vi "EventDetectionMode vol no 6230 DO.vi"(8 "error in (no error)":errorcluster, 11 "SetupInfo_IN":T1={"ConfigParameters_Analog"={"JAI camera fps"=240.0, "Bi-Lateral Galvo xy scan range (V)"=0.7, "Bi-Lateral Galvo xy scan frequency (Hz)"=500, "AOM Blind percent (%)"=0.1, "AOM start blind percent (%) "=70.0, "ROI threshold"=1.0, "AO Sampling rate"=1000000.0}, "ConfigParameters_Digital"={"Steps per volume"=25.0, "Time per volume (s)"=0.4, "OG start layer"=15.0, "Objective Lin Rising Vel (micron/ms）"=1.0, "Image depth (micron)"=200.0, "OG latency (s)"=10.0, "OG repitation"=3.0, "OG end layer"=17.0, "Shock1 duration (s)"=0.001, "Shock2 duration (s)"=0.001, "Shock3 duration (s)"=0.01, "Shock4 duration (s)"=0.01, "Shock5 duration (s)"=0.1, "Shock duration_New"=[]}, "ConfigParameters_Other1"={"Frontal Galvo xy scan range (V)"=0.14, "Frontal Galvo xy scan frequency (Hz)"=500, "PFI 0 digital clock frequency"=500000.0, "Window size for layer index"=0.5, "sCMOS fps"=95.0}, "ConfigParameters_Others2"={"#Trials baseline"=6, "#Trials test"=6, "Time before acq. (s)"=360.0, "Time before test (s)"=600.0, "#Blocks acquisition"=5, "Inter-trial interval baseline (s)"=60.0, "#Trials per acquition block"=6, "Inter-block interval acquisition (s)"=360.0, "Inter-trial interval acquisition (s)"=20.0, "Flash latency (s)"=10.0, "Flash duration (s)"=3.2, "Response duration (s)"=10.0, "MaxTimeEventDetection (s)"=6, "StimType"=enum."Flash", "#MaxEvents"=6}, "ProcessParametersOut"={"stand Z vol Acquisition time (s)"=0.2631578947368421, "stand Z vol Backward time (s)"=0.13684210526315793, "Objective scan volt"=5.0, "Bi-lateral Galvo Z scan volt"=0.1800000180000018, "Frontal Galvo Z scan volt"=0.14940000509752818, "Objective step length (micron)"=8.0, "OG Z volet Linear Dec time (s)"=0.024, "OG Z vol Stim. steps time (s)"=0.031578947368421054, "OG Z vol Linear Acc time (s)"=0.112, "#Vol. of flash"=8, "#Vol. of shock"=1, "#Vol. bef flash"=25, "#Vol. aft flash"=17, "OG Z vol Linear Dec time (s)"=0.112, "OG Z vol time (s)"=0.39073684210526316, "Stack duration"=[0.001, 0.001, 0.01, 0.01, 0.1], "AOM stand. value size"=400000, "Plane indexing length"=0, "#Vol. blank"=0, "#Vol. blank before acq"=1000000, "#Vol. blank before test"=263158, " #Inter-block interval acquisition (Ed-St Vol)"=1000000}, "WaveformParameters"={"stand Z vol Acquisition samp info"={"Fs"=1000000.0, "#s"=263158.0}, "stand Z vol Backward samp info"={"Fs"=1000000.0, "#s"=136842.0}, "OG Z vol Linear Acc samp info"={"Fs"=1000000.0, "#s"=112000.0}, "OG Z vol Stim. steps samp info"={"Fs"=1000000.0, "#s"=31579.0}, "OG Z volet Linear Dec samp info"={"Fs"=1000000.0, "#s"=24000.0}, "OG Z vol Linear Dec samp info"={"Fs"=1000000.0, "#s"=112000.0}, "OG Z vol samp info"={"Fs"=1000000.0, "#s"=390737.0}, "stand Z vol backforth samp info"={"Fs"=1000000.0, "#s"=400000.0}}, "AnalogWaveform"={"Bi-lateral Galvo Z stand waveform"={"t0"=timestamp(0 s since 1904-01-01), "dt"=1.0, "Y"=[]}, "Frontal Galvo Z stand waveform"={"t0"=timestamp(0 s since 1904-01-01), "dt"=1.0, "Y"=[]}, "Bi-lateral Galvo XY stand waveform"={"t0"=timestamp(0 s since 1904-01-01), "dt"=1.0, "Y"=[]}, "Frontal Galvo XY stand waveform"={"t0"=timestamp(0 s since 1904-01-01), "dt"=1.0, "Y"=[]}, "sCMOS stand waveform"={"t0"=timestamp(0 s since 1904-01-01), "dt"=1.0, "Y"=[]}, "Detection objective stand waveform"={"t0"=timestamp(0 s since 1904-01-01), "dt"=1.0, "Y"=[]}, "AOM stand waveform"={"t0"=timestamp(0 s since 1904-01-01), "dt"=1.0, "Y"=[]}, "PFI 0 clock stand waveform"={"t0"=timestamp(0 s since 1904-01-01), "dt"=1.0, "Y"=[]}, "Bi-lateral Galvo Z OG waveform"={"t0"=timestamp(0 s since 1904-01-01), "dt"=1.0, "Y"=[]}, "Bi-lateral Galvo XY OG waveform"={"t0"=timestamp(0 s since 1904-01-01), "dt"=1.0, "Y"=[]}, "Frontal Galvo Z OG waveform"={"t0"=timestamp(0 s since 1904-01-01), "dt"=1.0, "Y"=[]}, "Frontal Galvo XY OG waveform"={"t0"=timestamp(0 s since 1904-01-01), "dt"=1.0, "Y"=[]}, "sCMOS OG waveform"={"t0"=timestamp(0 s since 1904-01-01), "dt"=1.0, "Y"=[]}, "Detection objective OG waveform"={"t0"=timestamp(0 s since 1904-01-01), "dt"=1.0, "Y"=[]}, "AOM OG waveform"={"t0"=timestamp(0 s since 1904-01-01), "dt"=1.0, "Y"=[]}, "PFI 0 clock OG wavee"={"t0"=timestamp(0 s since 1904-01-01), "dt"=1.0, "Y"=[]}, "sCMOS blank waveform"={"t0"=timestamp(0 s since 1904-01-01), "dt"=1.0, "Y"=[]}, "All analog OG wave"=[], "All analog stand wave"=[], "All analog blank wave"=[], "BufferWaveform_Analog"=[], "Bi-lateral Galvo Z XY"={"t0"=timestamp(0 s since 1904-01-01), "dt"=1.0, "Y"=[]}, "Frontal Galvo Z XY"={"t0"=timestamp(0 s since 1904-01-01), "dt"=1.0, "Y"=[]}, "sCMOS Trigger XY"={"t0"=timestamp(0 s since 1904-01-01), "dt"=1.0, "Y"=[]}, "Detection objective XY"={"t0"=timestamp(0 s since 1904-01-01), "dt"=1.0, "Y"=[]}, "AOM XY"={"t0"=timestamp(0 s since 1904-01-01), "dt"=1.0, "Y"=[]}, "Analog_XY"=[]}, "DigitalWaveform"={"AllDigitalStandWave"=[], "AllDigialEvokedWave"=[], "AllDigialOGWave"=[], "AllDigitalPairWave_1"=[], "AllDigitalPairWave_2"=[], "AllDigitalPairWave_3"=[], "AllDigitalPairWave_4"=[], "AllDigitalPairWave_5"=[], "Plane Indexing"={"t0"=timestamp(0 s since 1904-01-01), "dt"=0.0, "Y"={"transitions"=[], "data"=[]}, "error"={"status"=FALSE, "code"=37421928, "source"=""}}, "Plane indexing P0.5 OG"={"t0"=timestamp(0 s since 1904-01-01), "dt"=0.0, "Y"={"transitions"=[], "data"=[]}, "error"={"status"=FALSE, "code"=37421928, "source"=""}}, "AllDigitalPairWaves"=[], "BufferWaveform_Digital"=[], "AllDigitalBlankWave"=[], "Digial_XY"=[], "Digital_XY_flash"=[], "Digial_XY DMD"=[]}, "PhysicalResource"={"PhysicalChannels_AI"="", "PhysicalChannels_AO"="", "PhysicalChannels_DO"="", "Task_AnalogOutput"="", "Task_DigitalOutput"="", "Task_AnalogInput"=""}, "ControlsRef"={"Mode_1"=refnum, "EventDetectionMode"=refnum, "Mode_2A"=refnum, "StimulationMode"=refnum, "Mode_2B"=refnum, "ErrorMeg"=refnum}, "test"=""} {"ConfigParameters_Other1"."Frontal Galvo xy scan frequency (Hz)" min=500 max=500; "ConfigParameters_Other1"."Frontal Galvo xy scan range (V)" min=0.0 max=1.5; "ConfigParameters_Analog"."AOM start blind percent (%)" min=10.0 max=90.0; "ConfigParameters_Analog"."AOM Blind percent (%)" min=0.1 max=100.0; "ConfigParameters_Analog"."Bi-Lateral Galvo xy scan frequency (Hz)" min=500 max=500; "ConfigParameters_Analog"."Bi-Lateral Galvo xy scan range (V)" min=0.0 max=1.5}) -> (0 "error out":errorcluster, 3 "SetupInfo_OUT":T1={"ConfigParameters_Analog"={"JAI camera fps"=240.0, "Bi-Lateral Galvo xy scan range (V)"=0.7, "Bi-Lateral Galvo xy scan frequency (Hz)"=500, "AOM Blind percent (%)"=0.1, "AOM start blind percent (%) "=70.0, "ROI threshold"=1.0, "AO Sampling rate"=1000000.0}, "ConfigParameters_Digital"={"Steps per volume"=25.0, "Time per volume (s)"=0.4, "OG start layer"=15.0, "Objective Lin Rising Vel (micron/ms）"=1.0, "Image depth (micron)"=200.0, "OG latency (s)"=10.0, "OG repitation"=3.0, "OG end layer"=17.0, "Shock1 duration (s)"=0.001, "Shock2 duration (s)"=0.001, "Shock3 duration (s)"=0.01, "Shock4 duration (s)"=0.01, "Shock5 duration (s)"=0.1, "Shock duration_New"=[]}, "ConfigParameters_Other1"={"Frontal Galvo xy scan range (V)"=0.14, "Frontal Galvo xy scan frequency (Hz)"=500, "PFI 0 digital clock frequency"=500000.0, "Window size for layer index"=0.5, "sCMOS fps"=95.0}, "ConfigParameters_Others2"={"#Trials baseline"=6, "#Trials test"=6, "Time before acq. (s)"=360.0, "Time before test (s)"=600.0, "#Blocks acquisition"=5, "Inter-trial interval baseline (s)"=60.0, "#Trials per acquition block"=6, "Inter-block interval acquisition (s)"=360.0, "Inter-trial interval acquisition (s)"=20.0, "Flash latency (s)"=10.0, "Flash duration (s)"=3.2, "Response duration (s)"=10.0, "MaxTimeEventDetection (s)"=6, "StimType"=enum."Flash", "#MaxEvents"=6}, "ProcessParametersOut"={"stand Z vol Acquisition time (s)"=0.2631578947368421, "stand Z vol Backward time (s)"=0.13684210526315793, "Objective scan volt"=5.0, "Bi-lateral Galvo Z scan volt"=0.1800000180000018, "Frontal Galvo Z scan volt"=0.14940000509752818, "Objective step length (micron)"=8.0, "OG Z volet Linear Dec time (s)"=0.024, "OG Z vol Stim. steps time (s)"=0.031578947368421054, "OG Z vol Linear Acc time (s)"=0.112, "#Vol. of flash"=8, "#Vol. of shock"=1, "#Vol. bef flash"=25, "#Vol. aft flash"=17, "OG Z vol Linear Dec time (s)"=0.112, "OG Z vol time (s)"=0.39073684210526316, "Stack duration"=[0.001, 0.001, 0.01, 0.01, 0.1], "AOM stand. value size"=400000, "Plane indexing length"=0, "#Vol. blank"=0, "#Vol. blank before acq"=1000000, "#Vol. blank before test"=263158, " #Inter-block interval acquisition (Ed-St Vol)"=1000000}, "WaveformParameters"={"stand Z vol Acquisition samp info"={"Fs"=1000000.0, "#s"=263158.0}, "stand Z vol Backward samp info"={"Fs"=1000000.0, "#s"=136842.0}, "OG Z vol Linear Acc samp info"={"Fs"=1000000.0, "#s"=112000.0}, "OG Z vol Stim. steps samp info"={"Fs"=1000000.0, "#s"=31579.0}, "OG Z volet Linear Dec samp info"={"Fs"=1000000.0, "#s"=24000.0}, "OG Z vol Linear Dec samp info"={"Fs"=1000000.0, "#s"=112000.0}, "OG Z vol samp info"={"Fs"=1000000.0, "#s"=390737.0}, "stand Z vol backforth samp info"={"Fs"=1000000.0, "#s"=400000.0}}, "AnalogWaveform"={"Bi-lateral Galvo Z stand waveform"={"t0"=timestamp(0 s since 1904-01-01), "dt"=1.0, "Y"=[]}, "Frontal Galvo Z stand waveform"={"t0"=timestamp(0 s since 1904-01-01), "dt"=1.0, "Y"=[]}, "Bi-lateral Galvo XY stand waveform"={"t0"=timestamp(0 s since 1904-01-01), "dt"=1.0, "Y"=[]}, "Frontal Galvo XY stand waveform"={"t0"=timestamp(0 s since 1904-01-01), "dt"=1.0, "Y"=[]}, "sCMOS stand waveform"={"t0"=timestamp(0 s since 1904-01-01), "dt"=1.0, "Y"=[]}, "Detection objective stand waveform"={"t0"=timestamp(0 s since 1904-01-01), "dt"=1.0, "Y"=[]}, "AOM stand waveform"={"t0"=timestamp(0 s since 1904-01-01), "dt"=1.0, "Y"=[]}, "PFI 0 clock stand waveform"={"t0"=timestamp(0 s since 1904-01-01), "dt"=1.0, "Y"=[]}, "Bi-lateral Galvo Z OG waveform"={"t0"=timestamp(0 s since 1904-01-01), "dt"=1.0, "Y"=[]}, "Bi-lateral Galvo XY OG waveform"={"t0"=timestamp(0 s since 1904-01-01), "dt"=1.0, "Y"=[]}, "Frontal Galvo Z OG waveform"={"t0"=timestamp(0 s since 1904-01-01), "dt"=1.0, "Y"=[]}, "Frontal Galvo XY OG waveform"={"t0"=timestamp(0 s since 1904-01-01), "dt"=1.0, "Y"=[]}, "sCMOS OG waveform"={"t0"=timestamp(0 s since 1904-01-01), "dt"=1.0, "Y"=[]}, "Detection objective OG waveform"={"t0"=timestamp(0 s since 1904-01-01), "dt"=1.0, "Y"=[]}, "AOM OG waveform"={"t0"=timestamp(0 s since 1904-01-01), "dt"=1.0, "Y"=[]}, "PFI 0 clock OG wavee"={"t0"=timestamp(0 s since 1904-01-01), "dt"=1.0, "Y"=[]}, "sCMOS blank waveform"={"t0"=timestamp(0 s since 1904-01-01), "dt"=1.0, "Y"=[]}, "All analog OG wave"=[], "All analog stand wave"=[], "All analog blank wave"=[], "BufferWaveform_Analog"=[], "Bi-lateral Galvo Z XY"={"t0"=timestamp(0 s since 1904-01-01), "dt"=1.0, "Y"=[]}, "Frontal Galvo Z XY"={"t0"=timestamp(0 s since 1904-01-01), "dt"=1.0, "Y"=[]}, "sCMOS Trigger XY"={"t0"=timestamp(0 s since 1904-01-01), "dt"=1.0, "Y"=[]}, "Detection objective XY"={"t0"=timestamp(0 s since 1904-01-01), "dt"=1.0, "Y"=[]}, "AOM XY"={"t0"=timestamp(0 s since 1904-01-01), "dt"=1.0, "Y"=[]}, "Analog_XY"=[]}, "DigitalWaveform"={"AllDigitalStandWave"=[], "AllDigialEvokedWave"=[], "AllDigialOGWave"=[], "AllDigitalPairWave_1"=[], "AllDigitalPairWave_2"=[], "AllDigitalPairWave_3"=[], "AllDigitalPairWave_4"=[], "AllDigitalPairWave_5"=[], "Plane Indexing"={"t0"=timestamp(0 s since 1904-01-01), "dt"=0.0, "Y"={"transitions"=[], "data"=[]}, "error"={"status"=FALSE, "code"=37421928, "source"=""}}, "Plane indexing P0.5 OG"={"t0"=timestamp(0 s since 1904-01-01), "dt"=0.0, "Y"={"transitions"=[], "data"=[]}, "error"={"status"=FALSE, "code"=37421928, "source"=""}}, "AllDigitalPairWaves"=[], "BufferWaveform_Digital"=[], "AllDigitalBlankWave"=[], "Digial_XY"=[], "Digital_XY_flash"=[], "Digial_XY DMD"=[]}, "PhysicalResource"={"PhysicalChannels_AI"="", "PhysicalChannels_AO"="", "PhysicalChannels_DO"="", "Task_AnalogOutput"="", "Task_DigitalOutput"="", "Task_AnalogInput"=""}, "ControlsRef"={"Mode_1"=refnum, "EventDetectionMode"=refnum, "Mode_2A"=refnum, "StimulationMode"=refnum, "Mode_2B"=refnum, "ErrorMeg"=refnum}, "test"=""} {"ConfigParameters_Other1"."Frontal Galvo xy scan frequency (Hz)" min=500 max=500; "ConfigParameters_Other1"."Frontal Galvo xy scan range (V)" min=0.0 max=1.5; "ConfigParameters_Analog"."AOM start blind percent (%)" min=10.0 max=90.0; "ConfigParameters_Analog"."AOM Blind percent (%)" min=0.1 max=100.0; "ConfigParameters_Analog"."Bi-Lateral Galvo xy scan frequency (Hz)" min=500 max=500; "ConfigParameters_Analog"."Bi-Lateral Galvo xy scan range (V)" min=0.0 max=1.5})   [LabVIEW 2018]
uses:
  SetupInfo.ctl
  ConfigParameters_Analog.ctl
  ConfigParameters_Digital.ctl
  ConfigParameters_Others1.ctl
  ConfigParameters_Others2.ctl
  ProcessParametersOut.ctl
  WaveformParameters.ctl
  AnalogWaveform.ctl
  DigitalWaveform.ctl
  PhysicalResource.ctl
  ControlsRef.ctl
  <vilib>/Analysis/baseanly.llb/Mean (DBL).vi
  Trigger_Global.vi
  <vilib>/Analysis/NI_AALBase.lvlib
panel:
  out "OG?":bool
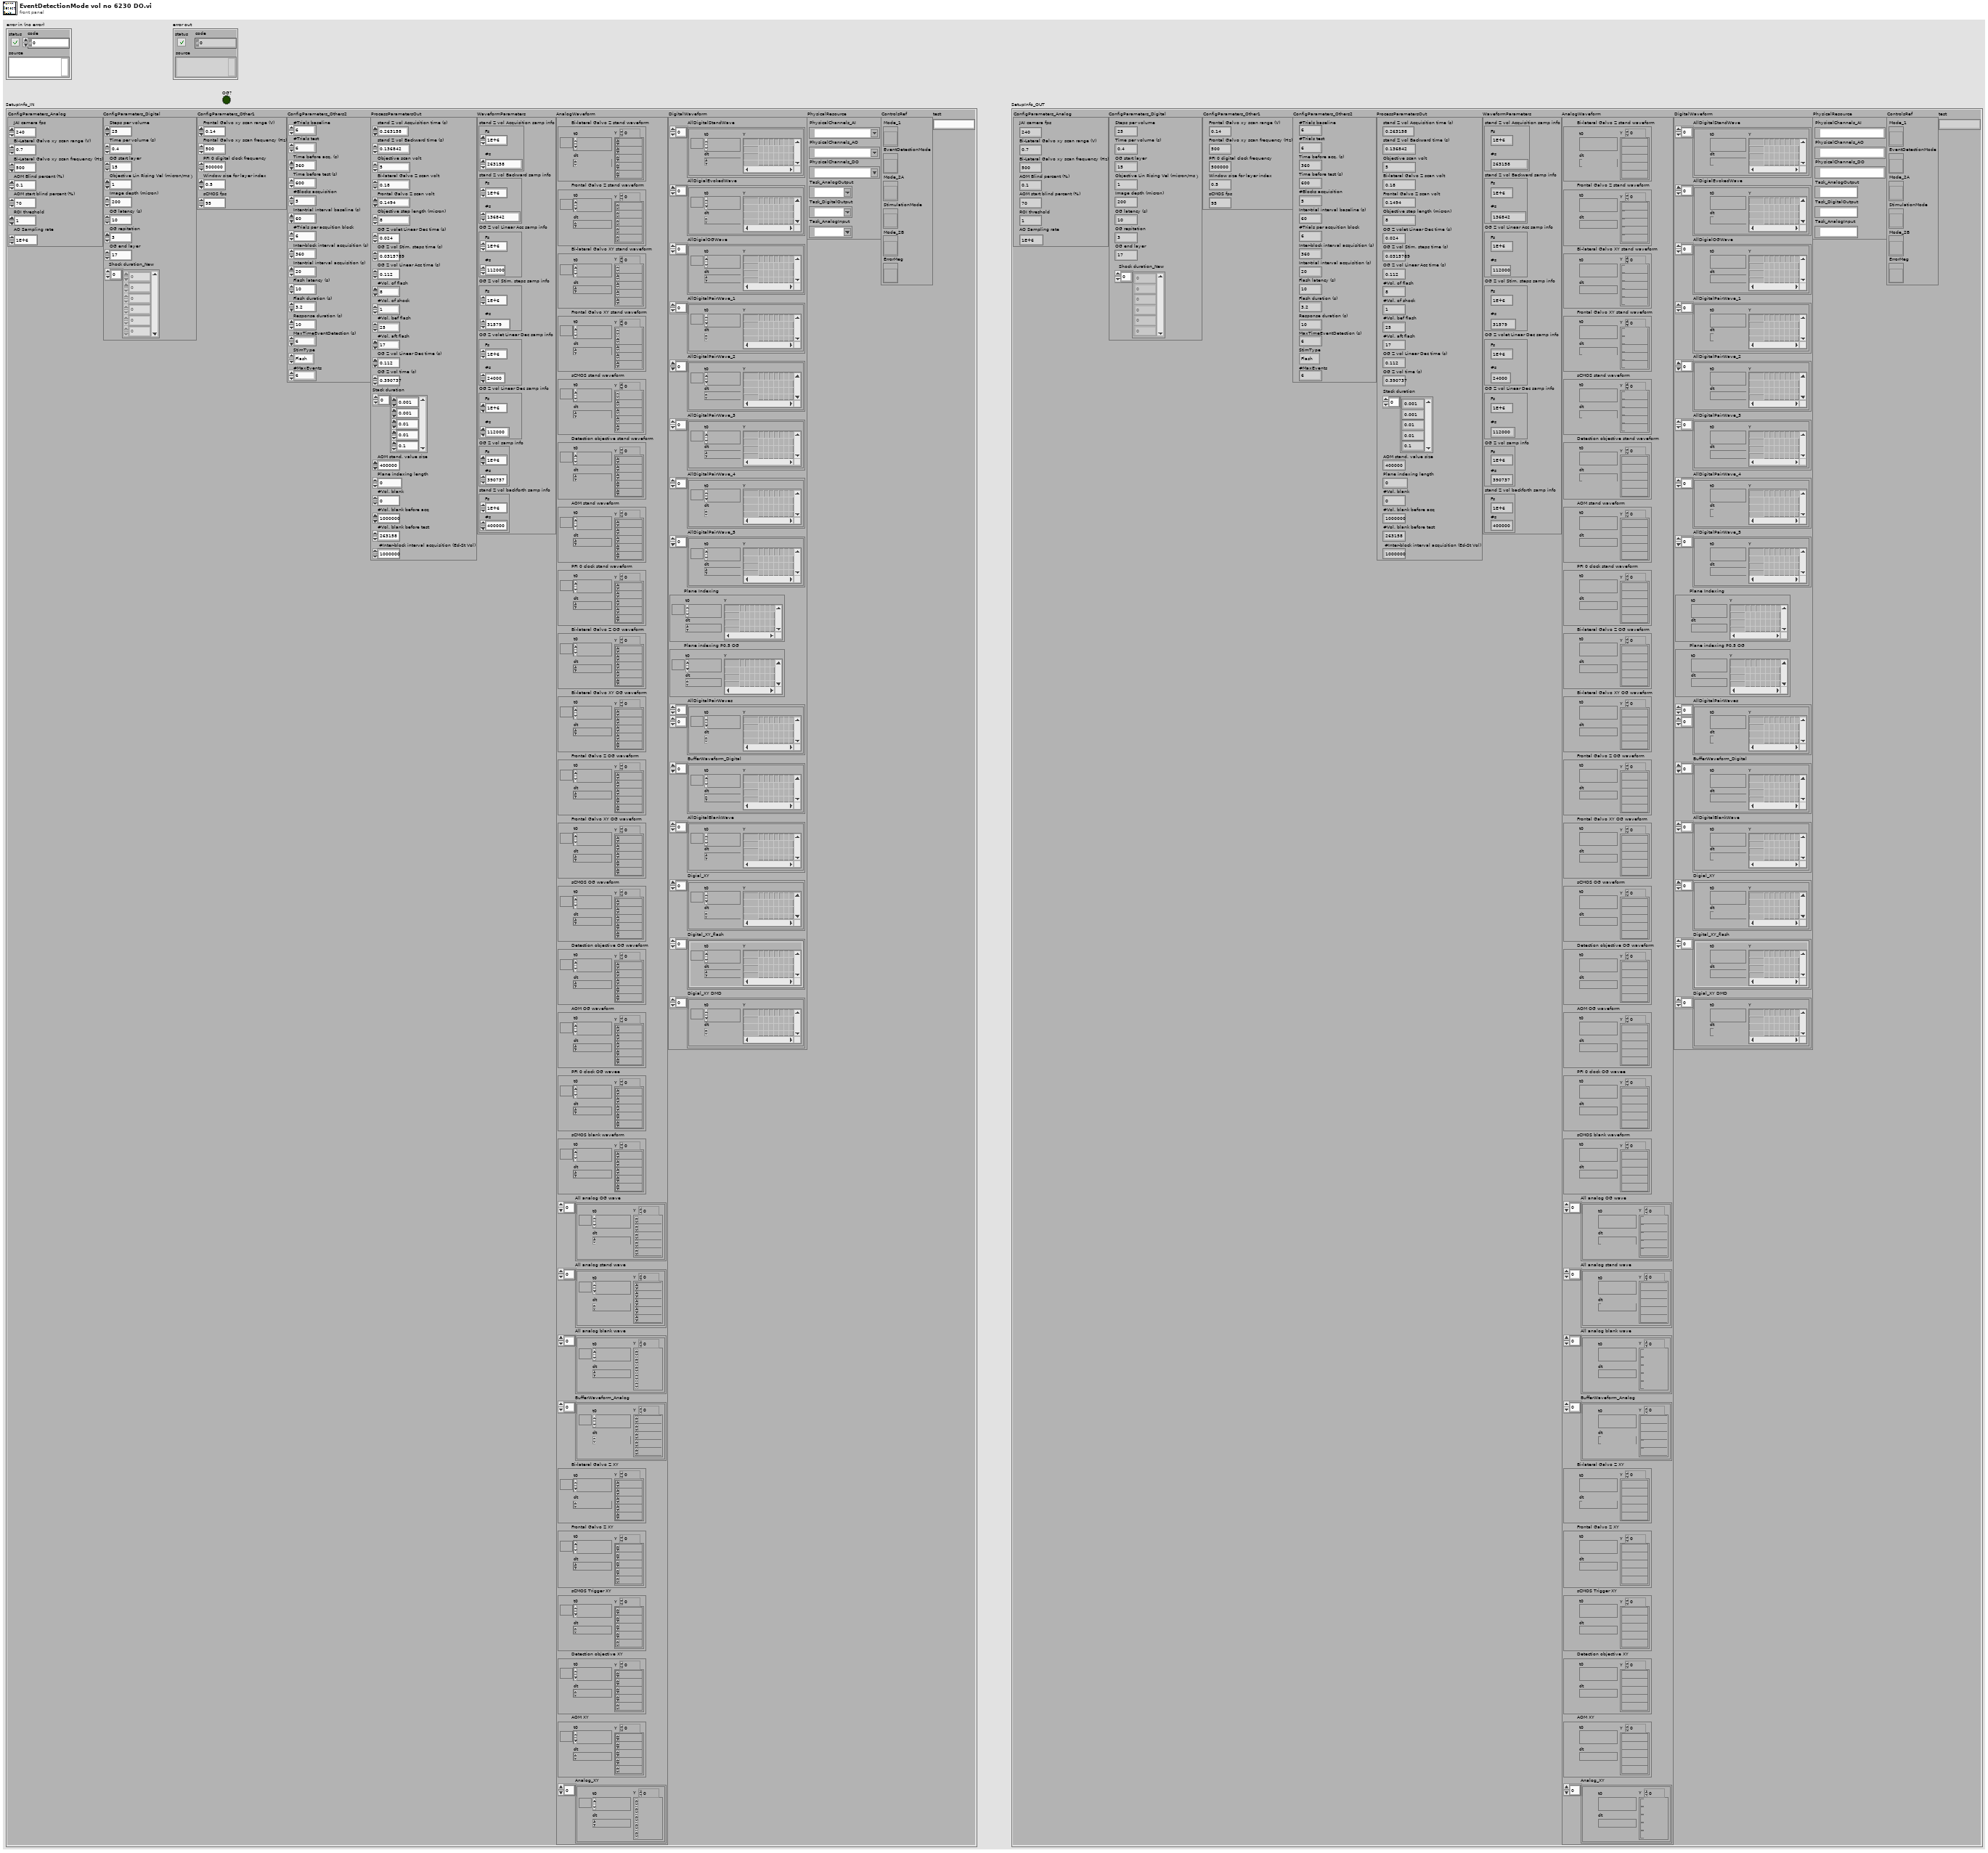
[diagram p1: front panel]
types:
  T1 = typedef "SetupInfo.ctl" = cluster{"ConfigParameters_Analog":T2, "ConfigParameters_Digital":T3, "ConfigParameters_Other1":T4, "ConfigParameters_Others2":T5, "ProcessParametersOut":T6, "WaveformParameters":T7, "AnalogWaveform":T8, "DigitalWaveform":T9, "PhysicalResource":T10, "ControlsRef":T11, "test":string}
  T2 = typedef "ConfigParameters_Analog.ctl" = cluster{"JAI camera fps":dbl, "Bi-Lateral Galvo xy scan range (V)":dbl, "Bi-Lateral Galvo xy scan frequency (Hz)":i16, "AOM Blind percent (%)":dbl, "AOM start blind percent (%) ":dbl, "ROI threshold":dbl, "AO Sampling rate":dbl}
  T3 = typedef "ConfigParameters_Digital.ctl" = cluster{"Steps per volume":dbl, "Time per volume (s)":dbl, "OG start layer":dbl, "Objective Lin Rising Vel (micron/ms）":dbl, "Image depth (micron)":dbl, "OG latency (s)":dbl, "OG repitation":dbl, "OG end layer":dbl, "Shock1 duration (s)":dbl, "Shock2 duration (s)":dbl, "Shock3 duration (s)":dbl, "Shock4 duration (s)":dbl, "Shock5 duration (s)":dbl, "Shock duration_New":dbl[]}
  T4 = typedef "ConfigParameters_Others1.ctl" = cluster{"Frontal Galvo xy scan range (V)":dbl, "Frontal Galvo xy scan frequency (Hz)":i16, "PFI 0 digital clock frequency":dbl, "Window size for layer index":dbl, "sCMOS fps":dbl}
  T5 = typedef "ConfigParameters_Others2.ctl" = cluster{"#Trials baseline":i32, "#Trials test":i32, "Time before acq. (s)":dbl, "Time before test (s)":dbl, "#Blocks acquisition":i32, "Inter-trial interval baseline (s)":dbl, "#Trials per acquition block":i32, "Inter-block interval acquisition (s)":dbl, "Inter-trial interval acquisition (s)":dbl, "Flash latency (s)":dbl, "Flash duration (s)":dbl, "Response duration (s)":dbl, "MaxTimeEventDetection (s)":i32, "StimType":enum16{"Flash", "OG"}, "#MaxEvents":i32}
  T6 = typedef "ProcessParametersOut.ctl" = cluster{"stand Z vol Acquisition time (s)":dbl, "stand Z vol Backward time (s)":dbl, "Objective scan volt":dbl, "Bi-lateral Galvo Z scan volt":dbl, "Frontal Galvo Z scan volt":dbl, "Objective step length (micron)":dbl, "OG Z volet Linear Dec time (s)":dbl, "OG Z vol Stim. steps time (s)":dbl, "OG Z vol Linear Acc time (s)":dbl, "#Vol. of flash":i32, "#Vol. of shock":i32, "#Vol. bef flash":i32, "#Vol. aft flash":i32, "OG Z vol Linear Dec time (s)":dbl, "OG Z vol time (s)":dbl, "Stack duration":dbl[], "AOM stand. value size":i32, "Plane indexing length":i32, "#Vol. blank":i32, "#Vol. blank before acq":i32, "#Vol. blank before test":i32, " #Inter-block interval acquisition (Ed-St Vol)":i32}
  T7 = typedef "WaveformParameters.ctl" = cluster{"stand Z vol Acquisition samp info":cluster{"Fs":dbl, "#s":dbl}, "stand Z vol Backward samp info":cluster{"Fs":dbl, "#s":dbl}, "OG Z vol Linear Acc samp info":cluster{"Fs":dbl, "#s":dbl}, "OG Z vol Stim. steps samp info":cluster{"Fs":dbl, "#s":dbl}, "OG Z volet Linear Dec samp info":cluster{"Fs":dbl, "#s":dbl}, "OG Z vol Linear Dec samp info":cluster{"Fs":dbl, "#s":dbl}, "OG Z vol samp info":cluster{"Fs":dbl, "#s":dbl}, "stand Z vol backforth samp info":cluster{"Fs":dbl, "#s":dbl}}
  T8 = typedef "AnalogWaveform.ctl" = cluster{"Bi-lateral Galvo Z stand waveform":waveform(dbl), "Frontal Galvo Z stand waveform":waveform(dbl), "Bi-lateral Galvo XY stand waveform":waveform(dbl), "Frontal Galvo XY stand waveform":waveform(dbl), "sCMOS stand waveform":waveform(dbl), "Detection objective stand waveform":waveform(dbl), "AOM stand waveform":waveform(dbl), "PFI 0 clock stand waveform":waveform(dbl), "Bi-lateral Galvo Z OG waveform":waveform(dbl), "Bi-lateral Galvo XY OG waveform":waveform(dbl), "Frontal Galvo Z OG waveform":waveform(dbl), "Frontal Galvo XY OG waveform":waveform(dbl), "sCMOS OG waveform":waveform(dbl), "Detection objective OG waveform":waveform(dbl), "AOM OG waveform":waveform(dbl), "PFI 0 clock OG wavee":waveform(dbl), "sCMOS blank waveform":waveform(dbl), "All analog OG wave":waveform(dbl)[], "All analog stand wave":waveform(dbl)[], "All analog blank wave":waveform(dbl)[], "BufferWaveform_Analog":waveform(dbl)[], "Bi-lateral Galvo Z XY":waveform(dbl), "Frontal Galvo Z XY":waveform(dbl), "sCMOS Trigger XY":waveform(dbl), "Detection objective XY":waveform(dbl), "AOM XY":waveform(dbl), "Analog_XY":waveform(dbl)[]}
  T9 = typedef "DigitalWaveform.ctl" = cluster{"AllDigitalStandWave":digitalwaveform[], "AllDigialEvokedWave":digitalwaveform[], "AllDigialOGWave":digitalwaveform[], "AllDigitalPairWave_1":digitalwaveform[], "AllDigitalPairWave_2":digitalwaveform[], "AllDigitalPairWave_3":digitalwaveform[], "AllDigitalPairWave_4":digitalwaveform[], "AllDigitalPairWave_5":digitalwaveform[], "Plane Indexing":digitalwaveform, "Plane indexing P0.5 OG":digitalwaveform, "AllDigitalPairWaves":digitalwaveform[][], "BufferWaveform_Digital":digitalwaveform[], "AllDigitalBlankWave":digitalwaveform[], "Digial_XY":digitalwaveform[], "Digital_XY_flash":digitalwaveform[], "Digial_XY DMD":digitalwaveform[]}
  T10 = typedef "PhysicalResource.ctl" = cluster{"PhysicalChannels_AI":tag, "PhysicalChannels_AO":tag, "PhysicalChannels_DO":tag, "Task_AnalogOutput":refnum<k21>, "Task_DigitalOutput":refnum<k21>, "Task_AnalogInput":refnum<k21>}
  T11 = typedef "ControlsRef.ctl" = cluster{"Mode_1":refnum<vi>, "EventDetectionMode":refnum<vi>, "Mode_2A":refnum<vi>, "StimulationMode":refnum<vi>, "Mode_2B":refnum<vi>, "ErrorMeg":refnum<vi>}
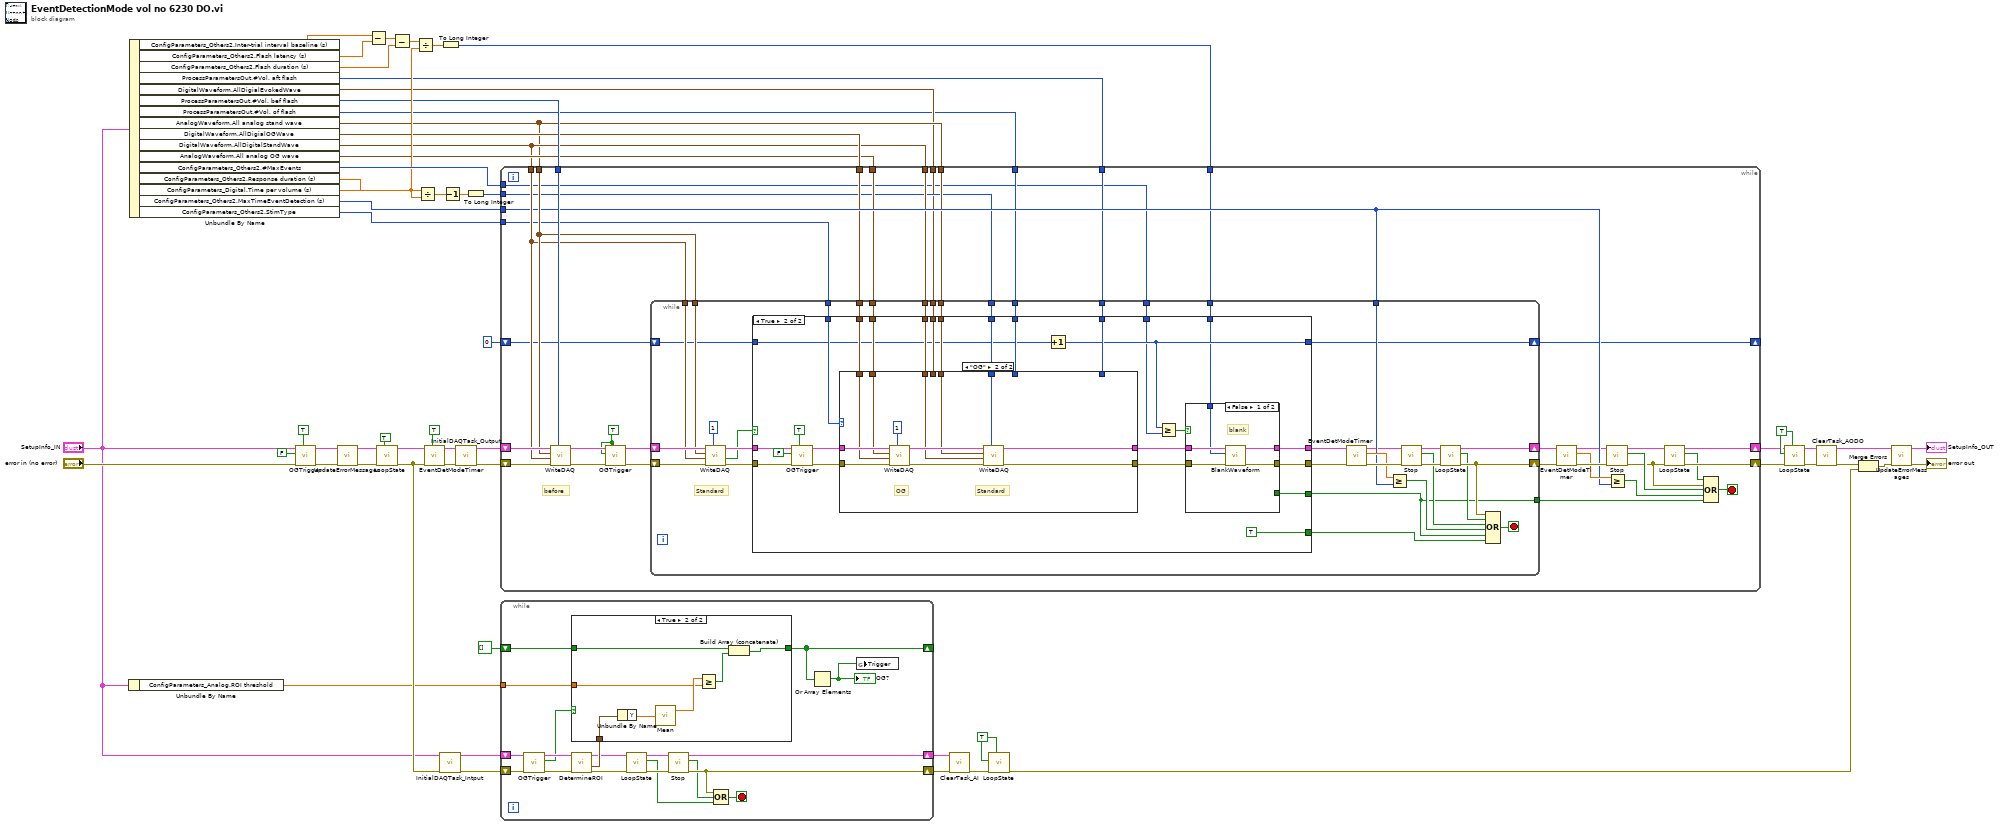
[diagram p0: block diagram]
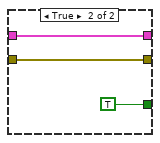
[diagram p3: hidden frame]
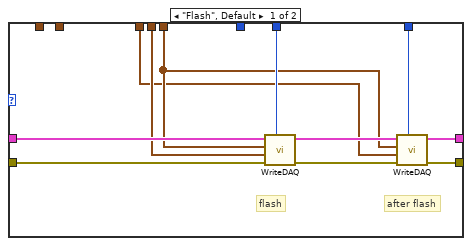
[diagram p4: hidden frame]
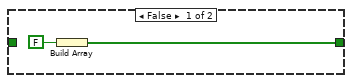
[diagram p5: hidden frame]
diagram:
  w41 = TRUE ("Write?")
  w49 = TRUE ("Write?")
  n1 = Unbundle By Name("SetupInfo_IN") -> ("ConfigParameters_Analog.ROI threshold"=w11:dbl)
  n2 = Unbundle By Name("SetupInfo_IN") -> ("ConfigParameters_Others2.Inter-trial interval baseline (s)"=w28:dbl, "ConfigParameters_Others2.Flash latency (s)"=w27:dbl, "ConfigParameters_Others2.Flash duration (s)"=w25:dbl, "ProcessParametersOut.#Vol. aft flash"=w3:i32, "DigitalWaveform.AllDigialEvokedWave"=w5:digitalwaveform[], "ProcessParametersOut.#Vol. bef flash"=w21:i32, "ProcessParametersOut.#Vol. of flash"=w4:i32, "AnalogWaveform.All analog stand wave"=w6:waveform(dbl)[], "DigitalWaveform.AllDigialOGWave"=w9:digitalwaveform[], "DigitalWaveform.AllDigitalStandWave"=w7:digitalwaveform[], "AnalogWaveform.All analog OG wave"=w8:waveform(dbl)[], "ConfigParameters_Others2.#MaxEvents"=w48:i32, "ConfigParameters_Others2.Response duration (s)"=w47:dbl, "ConfigParameters_Digital.Time per volume (s)"=w23:dbl, "ConfigParameters_Others2.MaxTimeEventDetection (s)"=w43:i32, "ConfigParameters_Others2.StimType"=w32:enum16{"Flash", "OG"})
  n3 = call "OGTrigger.vi"("Write?"=TRUE, "error in (no error)"="error in (no error)", "StateIn"=FALSE) -> ("error out"=w15:errorcluster)  [unwired: 7 in, 1 out]
  n4 = call "UpdateErrorMessages.vi"("error in (no error)"=w15, "SetupInfo_IN"="SetupInfo_IN") -> ("error out"=w33:errorcluster, "SetupInfo_OUT"=w34:T1)  [unwired: 8 in]
  n5 = Subtract(x=w28, y=w27) -> (x-y=w26:dbl)
  n6 = call "LoopState.vi"("Write?"=TRUE, "error in (no error)"=w33) -> ("error out"=w18:errorcluster)  [unwired: 8 in, 1 out]
  n7 = Subtract(x=w26, y=w25) -> (x-y=w24:dbl)
  n8 = Divide(x=w24, y=w23) -> (x/y=w22:dbl)
  n9 = Divide(x=w47, y=w23) -> (x/y=w46:dbl)
  n10 = call "EventDetModeTimer.vi"("Initial"=TRUE, "error in (no error)"=w18) -> ("error out"=w19:errorcluster)  [unwired: 8 in, 1 out]
  n11 = call "InitialDAQTask_Intput.vi"("error in (no error)"=w18, "SetupInfo_IN"="SetupInfo_IN") -> ("error out"=w55:errorcluster, "SetupInfo_OUT"=w42:T1)  [unwired: 8 in]
  n12 = To Long Integer(number=w22) -> (32bit integer=w2:i32)
  n13 = Decrement(x=w46) -> (x-1=w45:dbl)
  n14 = call "InitialDAQTask_Output.vi"("error in (no error)"=w19, "SetupInfo_IN"=w34) -> ("error out"=w17:errorcluster, "SetupInfo_OUT"=w20:T1)  [unwired: 8 in]
  n15 = To Long Integer(number=w45) -> (32bit integer=w31:i32)
  n16 = while {
    shift-right: [w83] -> w29
    shift-left: w17 -> [w80]
    shift-right: [w58] -> w30
    shift-left: w20 -> [w81]
    tunnel: w48 -> [w62]
    tunnel: w31 -> [w66]
    tunnel: w43 -> [w75]
    tunnel: w32 -> [w67]
    tunnel: w21 -> [w79]
    tunnel: w6 -> [w77]
    tunnel: w7 -> [w76]
    tunnel: w9 -> [w71]
    tunnel: w8 -> [w70]
    tunnel: w7 -> [w69]
    tunnel: w6 -> [w68]
    tunnel: w5 -> [w65]
    tunnel: w4 -> [w64]
    tunnel: w3 -> [w63]
    tunnel: w2 -> [w61]
    shift-right: [w60] -> _
    shift-left: 0 -> [w59]
    stop <- w87 stop-if-true
    w74 = TRUE ("Write?")
    # "before"
    n17 = call "WriteDAQ.vi"("Cycle"=w79, "error in (no error)"=w80, "DigitalWaveform_In"=w76, "AnalogWaveform_In"=w77, "SetupInfo_IN"=w81) -> ("error out"=w72:errorcluster, "SetupInfo_OUT"=w78:T1)  [unwired: 4 in, 1 out]
    n18 = call "OGTrigger.vi"("Write?"=w74, "error in (no error)"=w72, "StateIn"=w74) -> ("error out"=w73:errorcluster)  [unwired: 7 in, 1 out]
    n19 = while {
      shift-right: [w97] -> w58
      shift-left: w78 -> [w123]
      shift-right: [w115] -> w56
      shift-left: w73 -> [w111]
      tunnel: w77 -> [w122]
      tunnel: w76 -> [w121]
      tunnel: w75 -> [w116]
      tunnel: w71 -> [w109]
      tunnel: w70 -> [w108]
      tunnel: w69 -> [w106]
      tunnel: w68 -> [w105]
      tunnel: w67 -> [w104]
      tunnel: w66 -> [w103]
      tunnel: w65 -> [w102]
      tunnel: w64 -> [w101]
      tunnel: w63 -> [w100]
      shift-right: [w94] -> w60
      shift-left: w59 -> [w95]
      tunnel: w62 -> [w93]
      tunnel: w61 -> [w92]
      tunnel: [w91] -> w57
      stop <- w120 stop-if-true
      # "Standard"
      n20 = call "WriteDAQ.vi"("Cycle"=1, "error in (no error)"=w111, "DigitalWaveform_In"=w121, "AnalogWaveform_In"=w122, "SetupInfo_IN"=w123) -> ("error out"=w98:errorcluster, "Trigger"=w96:bool, "SetupInfo_OUT"=w107:T1)  [unwired: 4 in]
      n21 = case shown="True" w96 {
        tunnel: w109 -> [_ w151]
        tunnel: w108 -> [_ w150]
        tunnel: w107 -> [w125 w149]
        tunnel: w106 -> [_ w148]
        tunnel: w105 -> [_ w147]
        tunnel: w104 -> [_ w146]
        tunnel: w103 -> [_ w145]
        tunnel: w102 -> [_ w144]
        tunnel: w101 -> [_ w143]
        tunnel: w100 -> [_ w142]
        tunnel: [w126 w135] -> w99
        tunnel: w98 -> [w126 w129]
        tunnel: [w125 w136] -> w97
        tunnel: w95 -> [w124 w141]
        tunnel: [w124 w140] -> w94
        tunnel: w93 -> [_ w139]
        tunnel: w92 -> [_ w133]
        tunnel: [_ w132] -> w91
        tunnel: [_ TRUE] -> w90
        frame False {
        }
        frame True {
          n22 = call "OGTrigger.vi"("Write?"=TRUE, "error in (no error)"=w129, "StateIn"=FALSE) -> ("error out"=w128:errorcluster)  [unwired: 7 in, 1 out]
          n23 = case shown="\"OG\"" w146 {
            tunnel: w128 -> [w169 w182]
            tunnel: w149 -> [w170 w181]
            tunnel: [w164 w172] -> w138
            tunnel: [w163 w171] -> w137
            tunnel: w150 -> [_ w180]
            tunnel: w151 -> [_ w179]
            tunnel: w147 -> [w161 w175]
            tunnel: w144 -> [w168 _]
            tunnel: w145 -> [_ w173]
            tunnel: w148 -> [w160 w174]
            tunnel: w143 -> [w167 _]
            tunnel: w142 -> [w162 _]
            frame "Flash", Default {
              # "after flash"
              # "flash"
              n24 = call "WriteDAQ.vi"("Cycle"=w167, "error in (no error)"=w169, "DigitalWaveform_In"=w168, "AnalogWaveform_In"=w161, "SetupInfo_IN"=w170) -> ("error out"=w165:errorcluster, "SetupInfo_OUT"=w166:T1)  [unwired: 4 in, 1 out]
              n25 = call "WriteDAQ.vi"("Cycle"=w162, "error in (no error)"=w165, "DigitalWaveform_In"=w160, "AnalogWaveform_In"=w161, "SetupInfo_IN"=w166) -> ("error out"=w163:errorcluster, "SetupInfo_OUT"=w164:T1)  [unwired: 4 in, 1 out]
            }
            frame "OG" {
              # "Standard"
              # "OG"
              n26 = call "WriteDAQ.vi"("Cycle"=1, "error in (no error)"=w182, "DigitalWaveform_In"=w179, "AnalogWaveform_In"=w180, "SetupInfo_IN"=w181) -> ("error out"=w176:errorcluster, "SetupInfo_OUT"=w177:T1)  [unwired: 4 in, 1 out]
              n27 = call "WriteDAQ.vi"("Cycle"=w173, "error in (no error)"=w176, "DigitalWaveform_In"=w174, "AnalogWaveform_In"=w175, "SetupInfo_IN"=w177) -> ("error out"=w171:errorcluster, "SetupInfo_OUT"=w172:T1)  [unwired: 4 in, 1 out]
            }
          }
          n28 = Increment(x=w141) -> (x+1=w140:i32)
          n29 = Greater Or Equal?(x=w140, y=w139) -> (x >= y?=w134:bool)
          n30 = case shown="False" w134 {
            tunnel: w137 -> [w156 w158]
            tunnel: w138 -> [w155 w159]
            tunnel: [w154 w159] -> w136
            tunnel: [w153 w158] -> w135
            tunnel: w133 -> [w152 _]
            tunnel: [_ TRUE] -> w132
            frame False {
              # "blank"
              n31 = call "BlankWaveform.vi"("error in (no error)"=w156, "Cycle"=w152, "SetupInfo_IN"=w155) -> ("error out"=w153:errorcluster, "SetupInfo_OUT"=w154:T1)  [unwired: 7 in]
            }
            frame True {
            }
          }
        }
      }
      n32 = call "EventDetModeTimer.vi"("error in (no error)"=w99) -> ("error out"=w118:errorcluster, "TimerOut(s)"=w117:dbl)  [unwired: 9 in]
      n33 = Greater Or Equal?(x=w117, y=w116) -> (x >= y?=w112:bool)
      n34 = call "Stop.vi"("error in (no error)"=w118) -> ("error out"=w119:errorcluster, "StateOut"=w113:bool)  [unwired: 9 in]
      n35 = call "LoopState.vi"("error in (no error)"=w119) -> ("error out"=w115:errorcluster, "StateOut"=w114:bool)  [unwired: 9 in]
      n36 = Compound Arithmetic op=OR(w115, w114, w113, w112, w91, w90) -> (w120:bool)
    }
    n37 = call "EventDetModeTimer.vi"("error in (no error)"=w56) -> ("error out"=w88:errorcluster, "TimerOut(s)"=w86:dbl)  [unwired: 9 in]
    n38 = call "Stop.vi"("error in (no error)"=w88) -> ("error out"=w84:errorcluster, "StateOut"=w89:bool)  [unwired: 9 in]
    n39 = Greater Or Equal?(x=w86, y=w75) -> (x >= y?=w85:bool)
    n40 = call "LoopState.vi"("error in (no error)"=w84) -> ("error out"=w83:errorcluster, "StateOut"=w82:bool)  [unwired: 9 in]
    n41 = Compound Arithmetic op=OR(w82, w84, w89, w85, w57) -> (w87:bool)
  }
  n42 = while {
    shift-right: [w198] -> w54
    shift-left: w55 -> [w190]
    shift-right: [w192] -> w53
    shift-left: w42 -> [w188]
    shift-right: [w185] -> _
    shift-left: bool[] [] -> [w187]
    tunnel: w11 -> [w186]
    stop <- w196 stop-if-true
    n43 = call "OGTrigger.vi"("error in (no error)"=w190) -> ("error out"=w191:errorcluster, "StateOut"=w184:bool)  [unwired: 9 in]
    n44 = call "DetermineROI.vi"("error in (no error)"=w191, "SetupInfo_IN"=w188) -> ("error out"=w189:errorcluster, "data"=w193:waveform(dbl), "SetupInfo_OUT"=w192:T1)  [unwired: 7 in]
    n45 = case shown="True" w184 {
      tunnel: w193 -> [_ w201]
      tunnel: [w199 w202] -> w185
      tunnel: w187 -> [_ w205]
      tunnel: w186 -> [_ w203]
      frame False {
        n46 = Build Array(FALSE) -> (w199:bool[])
      }
      frame True {
        n47 = Unbundle By Name(w201) -> ("Y"=w206:dbl[])
        n48 = call-poly <vilib>:"Mean.vi"("X"=w206) -> ("mean"=w207:dbl)  [unwired: 1 out]
        n49 = Greater Or Equal?(x=w207, y=w203) -> (x >= y?=w204:bool)
        n50 = Build Array (concatenate)(w205, w204) -> (w202:bool[])
      }
    }
    n51 = call "LoopState.vi"("error in (no error)"=w189) -> ("error out"=w195:errorcluster, "StateOut"=w194:bool)  [unwired: 9 in]
    n52 = call "Stop.vi"("error in (no error)"=w195) -> ("error out"=w198:errorcluster, "StateOut"=w197:bool)  [unwired: 9 in]
    n53 = Compound Arithmetic op=OR(w198, w197, w194) -> (w196:bool)
    n54 = Or Array Elements(Boolean array=w185) -> (logical OR=w183:bool)
    "OG?" <- w183
    n55 = global write "Trigger_Global.vi" "Trigger"(w183) -> ()
  }
  n56 = call "ClearTask_AI.vi"("error in (no error)"=w54, "SetupInfo_IN"=w53) -> ("error out"=w40:errorcluster)  [unwired: 8 in, 1 out]
  n57 = call "LoopState.vi"("Write?"=w41, "error in (no error)"=w40, "StateIn"=w41) -> ("error out"=w39:errorcluster)  [unwired: 7 in, 1 out]
  n58 = call "LoopState.vi"("Write?"=w49, "error in (no error)"=w29, "StateIn"=w49) -> ("error out"=w50:errorcluster)  [unwired: 7 in, 1 out]
  n59 = call "ClearTask_AODO.vi"("error in (no error)"=w50, "SetupInfo_IN"=w30) -> ("error out"=w52:errorcluster, "SetupInfo_OUT"=w37:T1)  [unwired: 8 in]
  n60 = Merge Errors(w52, w39) -> (w38:errorcluster)
  n61 = call "UpdateErrorMessages.vi"("error in (no error)"=w38, "SetupInfo_IN"=w37) -> ("error out"=→"error out":errorcluster, "SetupInfo_OUT"=→"SetupInfo_OUT":T1)  [unwired: 8 in]
